vi "add_visa_out_error_out.vi"(0 "VI Ref In":refnum<vi>, 5 "Visa Out  Position":cluster{"Left":u32, "Top":i32}, 7 "Error Out  Position":cluster{"Left":u32, "Top":i32}, 11 "error in":errorcluster) -> (4 "VI Ref Out":refnum<vi>, 6 "Visa Out Term":refnum<vi>, 8 "Error Out Term":refnum<vi>, 15 "error out":errorcluster)   [LabVIEW 2018]
uses:
  Iternl/AddObj/AddControl/TypeDefinitions/bd_control_type.ctl
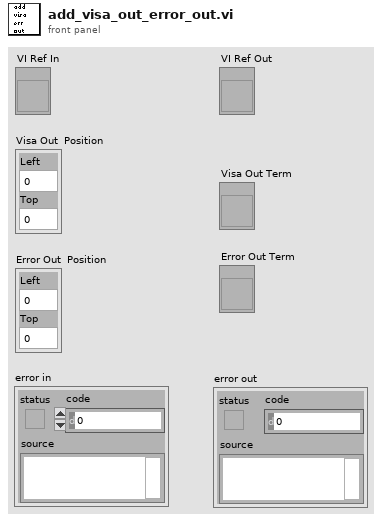
[diagram p1: front panel]
types:
  T1 = typedef "bd_control_type.ctl" = enum16{"Numeric", "Ring", "Boolean", "String", "VisaIn", "VisaOut", "Error In", "Error Out", "Array", "Waveform"}
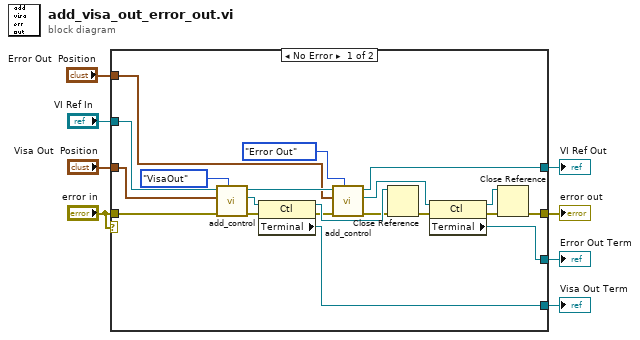
[diagram p0: block diagram]
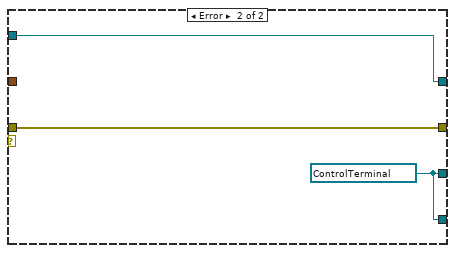
[diagram p2: hidden frame]
diagram:
  n1 = case shown="No Error" "error in" {
    tunnel: "error in" -> [w26 w31]
    tunnel: "VI Ref In" -> [w25 w29]
    tunnel: "Error Out  Position" -> [w24 _]
    tunnel: [w22 w29] -> w6
    tunnel: [w17 w30] -> w5
    tunnel: [w16 w30] -> w4
    tunnel: "Visa Out  Position" -> [w15 _]
    tunnel: [w11 w31] -> w2
    frame No Error {
      n2 = call "add_control.vi"("Add Control Type"=bd_control_type."VisaOut" ("Enum"), "error in (no error)"=w26, "BD Position"=w15, "VI Ref In"=w25) -> ("error out"=w14:errorcluster, "Control Ref Out"=w23:refnum<vi>, "VI Ref Out"=w27:refnum<vi>)  [unwired: 1 in, 4 out]
      n3 = property class="Ctl"(reference=w23, error in=w14) -> (reference out=w20:refnum<vi>, error out=w10:errorcluster, "Terminal"=w16:refnum<vi>)
      n4 = call "add_control.vi"("Add Control Type"=bd_control_type."Error Out" ("Enum"), "error in (no error)"=w10, "BD Position"=w24, "VI Ref In"=w27) -> ("error out"=w9:errorcluster, "Control Ref Out"=w21:refnum<vi>, "VI Ref Out"=w22:refnum<vi>)  [unwired: 1 in, 4 out]
      n5 = Close Reference(reference=w20, error in (no error)=w9) -> (error out=w28:errorcluster)
      n6 = property class="Ctl"(reference=w21, error in=w28) -> (reference out=w19:refnum<vi>, error out=w18:errorcluster, "Terminal"=w17:refnum<vi>)
      n7 = Close Reference(reference=w19, error in (no error)=w18) -> (error out=w11:errorcluster)
    }
    frame Error {
      w30 = refnum<vi> refnum ("Terminal")
    }
  }
  "VI Ref Out" <- w6
  "Error Out Term" <- w5
  "Visa Out Term" <- w4
  "error out" <- w2
